vi "Datestring (SubVI).vi"() -> (3 "datestring":string)   [LabVIEW 2020, in "FileIO.lvlib"]
uses:
  FileIO.lvlib
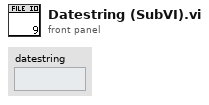
[diagram p1: front panel]
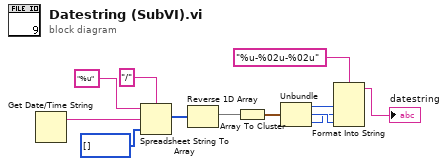
[diagram p0: block diagram]
diagram:
  n1 = Get Date/Time String() -> (date string=w10:string)  [unwired: 3 in, 1 out]
  n2 = Spreadsheet String To Array(delimiter (Tab)="/", format string="%u", spreadsheet string=w10, array type (2D Dbl)=u16[] []) -> (array=w8:u16[])
  n3 = Reverse 1D Array(array=w8) -> (reversed array=w7:u16[])
  n4 = Array To Cluster(array=w7) -> (cluster=w6:cluster{"[0]":u16, "[1]":u16, "[2]":u16})
  n5 = Unbundle(w6) -> ("[0]"=w5:u16, "[1]"=w2:u16, "[2]"=w1:u16)
  n6 = Format Into String(format string="%u-%02u-%02u", w5, w1, w2) -> (resulting string=→"datestring":string)  [unwired: 2 in, 1 out]
